vi "ReadISOStatus.vi"(6 "time out":u32, 10 "类型":u32(ring)=4 items=["PCI5121"=1, "PCI9810"=2, "USBCAN1"=3, "USBCAN2"=4, "PCI9820"=5, "CAN232"=6, "PCI5110"=7, "CANLite(mini)"=8, "ISA9620"=9, "ISA5420"=10, "PC104CAN"=11, "CANET"=17, "DNP9810"=13, "USBCAN-E-U"=20, "USBCAN-2E-U"=21], 12 "设备索引":u32(ring) items=["0", "1", "2", "3", "4", "5", "6", "7", "8", "9", "10", "11", "12", "13", "14", "15", ""], 16 "CAN路数":u32(ring) items=["0", "1"]) -> (20 "recv ok?":bool, 22 "ISO":i8)   [LabVIEW 2013]
uses:
  AutoBurn/Settings/ControlCAN.dll
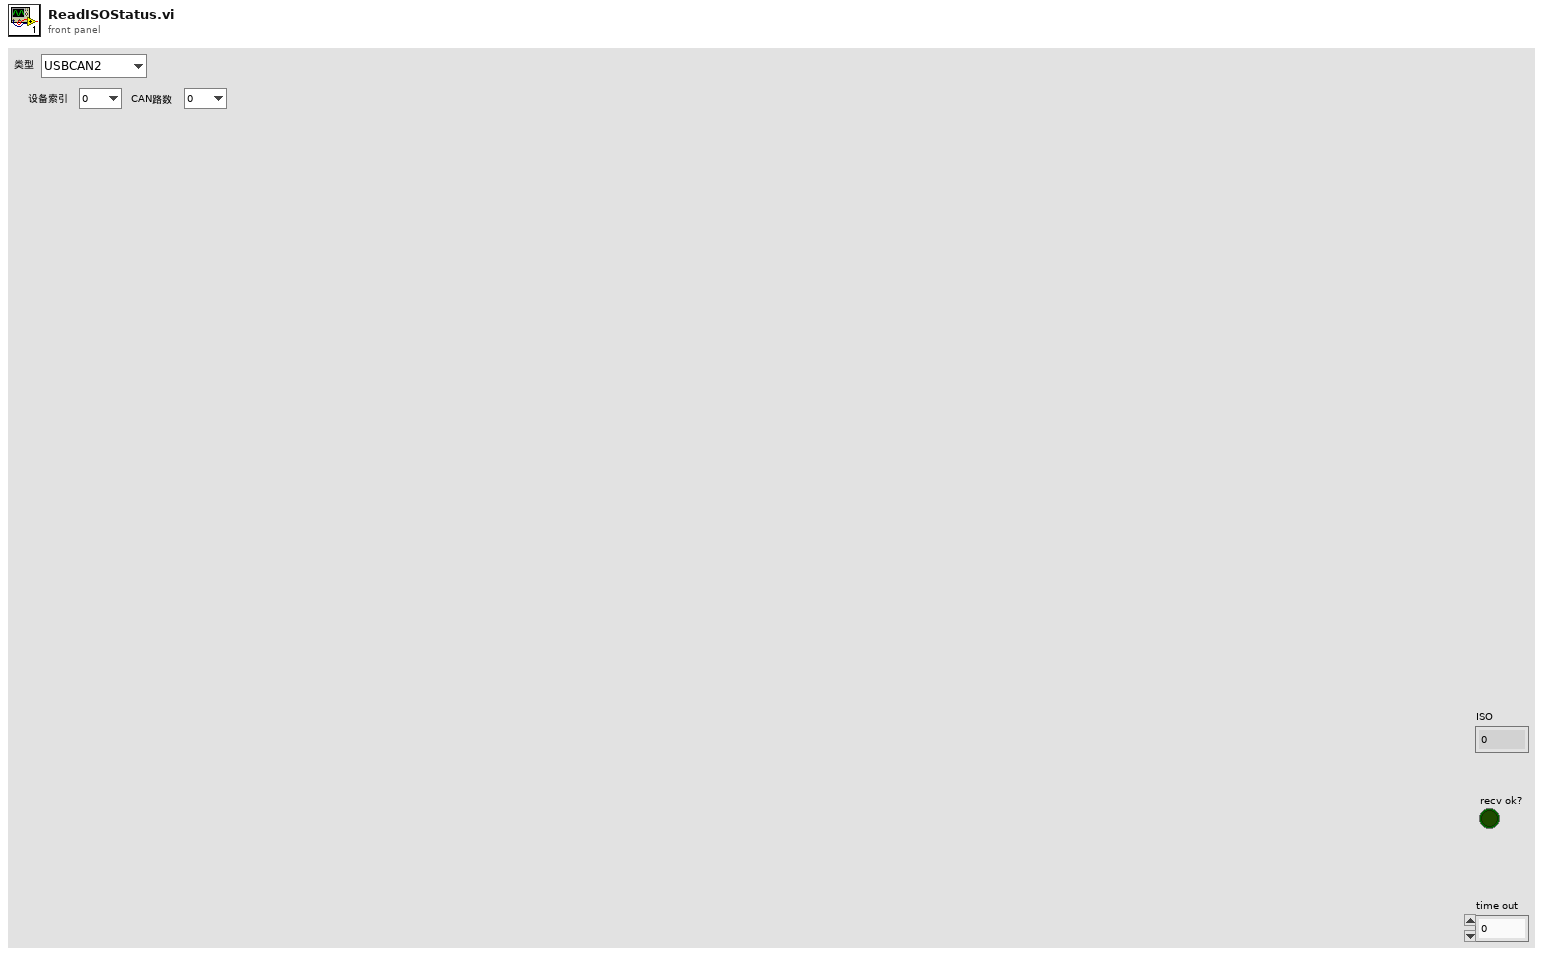
[diagram p1: front panel]
types:
  T1 = cluster{"ID":u32, "TimeStamp":u32, "TimeFlag":u8, "SendType":u8, "RemoteFlag":u8, "ExternFlag":u8, "DataLen":u8, u8, u8, u8, u8, u8, u8, u8, u8, u8, u8, u8}
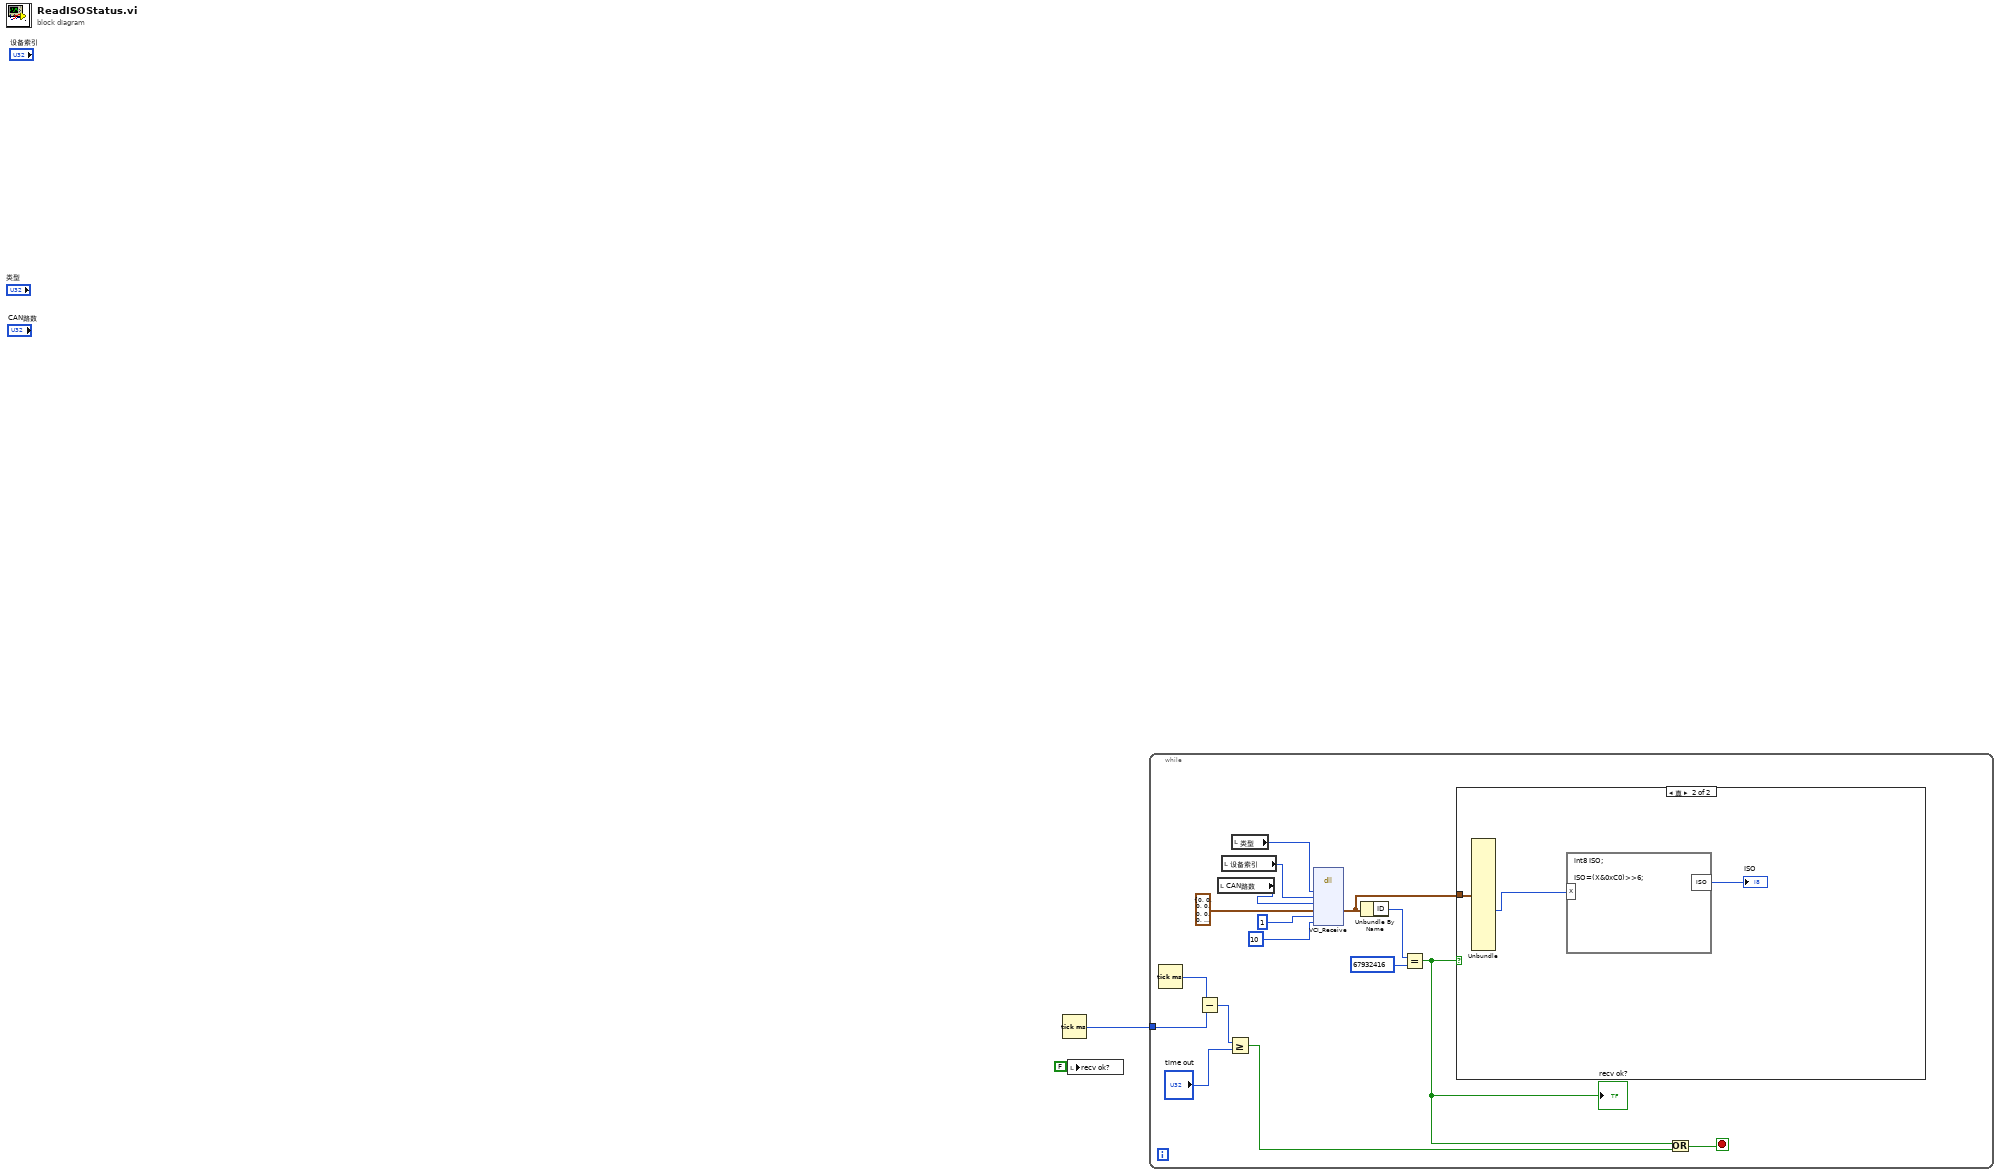
[diagram p0: block diagram]
diagram:
  n1 = Tick Count (ms)() -> (millisecond timer value=w2:u32)
  n2 = local write "recv ok?"(FALSE ("x = y?")) -> ()
  n3 = while {
    tunnel: w2 -> [w11]
    stop <- w5 stop-if-true
    n4 = Tick Count (ms)() -> (millisecond timer value=w12:u32)
    n5 = Subtract(x=w12, y=w11) -> (x-y=w10:u32)
    n6 = local read "CAN路数"() -> (w16:u32)
    n7 = local read "设备索引"() -> (w13:u32)
    n8 = Greater Or Equal?(x=w10, y="time out") -> (x >= y?=w6:bool)
    n9 = local read "类型"() -> (w14:u32)
    n10 = dll-call lib="F:/Bluewave New Energy/SVN_Work/AutoTest_TestStand/trunk/AutoTest_TestStand/Driver/ZlgCan/BHN01/AutoBurn/Settings/ControlCAN.dll" fn="VCI_Receive"("DeviceType"=w14, "DeviceInd"=w13, "CANInd"=w16, "pReceive"=T1 {"ID"=0, "TimeStamp"=0, "TimeFlag"=0, "SendType"=0, "RemoteFlag"=0, "ExternFlag"=0, "DataLen"=0, 0, 0, 0, 0, 0, 0, 0, 0, 0, 0, 0}, "Len"=u32 1, "WaitTime"=10) -> ("pReceive"=w4:T1)  [unwired: 8 in, 3 out]
    n11 = Unbundle By Name(w4) -> ("ID"=w8:u32)
    n12 = Equal?(x=w8, y=u32 67932416) -> (x = y?=w7:bool)
    "recv ok?" <- w7
    n13 = case shown="真" w7 {
      tunnel: w4 -> [_ w21]
      frame False {
      }
      frame True {
        n14 = Unbundle(w21) -> (w19:u8)  [unwired: 17 out]
        n15 = formula code="int8 ISO;\n\nISO=(X&0xC0)>>6;"("X"=w19) -> ("ISO"=→"ISO":i8)
      }
    }
    n16 = Or(x=w7, y=w6) -> (x .or. y?=w5:bool)
  }
